vi "Wyznaczanie promienia krzywizny (parametr c).vi"(4 "Parametry Ziemi":T1={"a - półoś duża"=6378137.0, "b - półoś mała"=6356752.3141999999998} {"b - półoś mała" format="%_20f"; "a - półoś duża" format="%_20g"}) -> (1 "c- promień krzywizny":ext=6378137.0 format="%_20g")   [LabVIEW 2015, in "Biblioteka moduł map v3.lvlib" / "Konwersja wsp.lvlib" / "UTM.lvlib"]
uses:
  UTM.lvlib
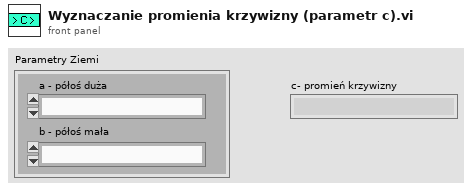
[diagram p1: front panel]
types:
  T1 = cluster{"a - półoś duża":ext, "b - półoś mała":ext}
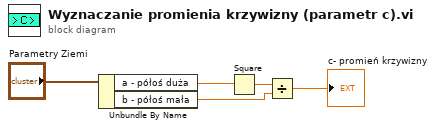
[diagram p0: block diagram]
diagram:
  n1 = Unbundle By Name("Parametry Ziemi") -> ("a - półoś duża"=w4:ext, "b - półoś mała"=w2:ext)
  n2 = Square(x=w4) -> (x^2=w3:ext)
  n3 = Divide(x=w3, y=w2) -> (x/y=→"c- promień krzywizny":ext)
